vi "One shot TCP AI.vi"() -> ()   [LabVIEW 2010]
uses:
  Send 1 Scan multi-channel.vi
  scale.ctl
  DAQ configuration/channel identifier.ctl
panel:
  in  "Reset graph":bool
  in  "history length":u16=1000 min=1
  out "XY Graph":cluster{dbl[], dbl[]}[](graph)
  out "Range error":bool[](array[boolean])
  out "units":string[](array[string])
  out "Scaled data":sgl[](array[numeric]) format="%.2f"
  out "voltage date":sgl[](array[numeric]) format="%.5f"
  in  "Scale type":T1[](array[typedef]) items=["200 kPa - cm", "200 kPa - orifice 1.6 mm", "200 kPa - orifice 3.2 mm", "200 kPa - Pa", "7 kPa - 1.5 cm vol det", "7 kPa - 10 cm vol det", "7 kPa - cm", "7 kPa - orifice 1.6 mm", "7 kPa - orifice 3.2 mm", "7 kPa - Pa", "7 kPa - Reservoir", "Thermistors - C1", "Thermistors - C2", "Thermistors - C3", "Thermistors - C4", "Thermistors - C5", "Thermistors - C6", "Thermistors - C7"]
  in  "Port":T2[](array[typedef])
  out "arbitrary time (s)":dbl format="%.2f"
  in  "millisecond multiple":u32
  in  "stop":bool
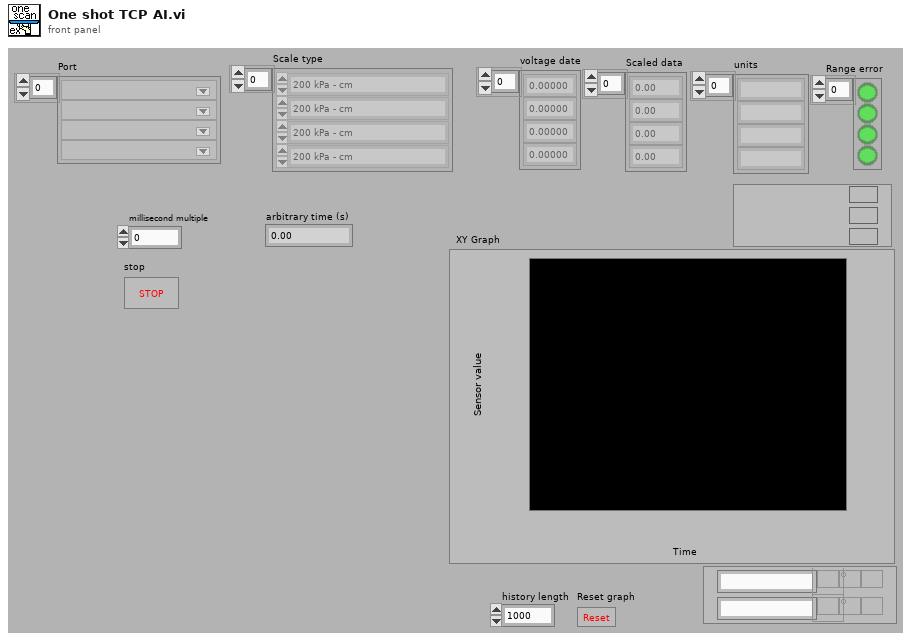
[diagram p1: front panel]
types:
  T1 = typedef "scale.ctl" = u16
  T2 = typedef "channel identifier.ctl" = u16
  T3 = cluster{"scan rate":dbl, "# connections":i32, "channels (0)":string[], "group channel settings":cluster{"channel":string, "upper input limits":sgl, "lower input limits":sgl, "range":sgl, "polarity":enum16{"no change", "bipolar", "unipolar"}, "gain":sgl, "coupling":enum16{"no change", "DC", "AC", "ground", "internal reference"}, "input mode":enum16{"no change", "differential", "rse", "nrse"}, "scale multiplier":sgl, "scale offset":sgl}[]}
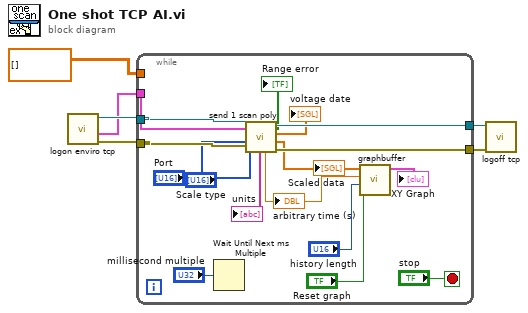
[diagram p0: block diagram]
diagram:
  n1 = call "logon enviro tcp.vi"(1:w2) -> ("error out"=w4:errorcluster, "connection ID"=w5:refnum<k5>)  [unwired: 8 in, 1 out]
  n2 = while {
    tunnel: [w16] -> w2
    tunnel: sgl[][] [] ("History Data") -> [_]
    tunnel: [w18] -> w3
    tunnel: w4 -> [w21]
    tunnel: w5 -> [w22]
    tunnel: [w23] -> w6
    stop <- "stop" stop-if-true
    n3 = Wait Until Next ms Multiple(millisecond multiple="millisecond multiple") -> ()  [unwired: 1 out]
    n4 = call-poly "send 1 scan poly.vi"("error in (no error)"=w21, "Scale type"="Scale type", "Port"="Port", "Connection ID in"=w22) -> ("error out"=w23:errorcluster, "Scaled data"=w10:sgl[], "voltage data"=→"voltage date":sgl[], "Connection ID out"=w18:refnum<k5>, "arbitrary time (s)"=w17:dbl, "Out of Range"=→"Range error":bool[], "units"=→"units":string[], "Server Stats"=w16:T3)
    "arbitrary time (s)" <- w17
    "Scaled data" <- w10
    n5 = call "graphbuffer.vi"("Reset"="Reset graph", "history length"="history length", "Time"=w17, "data"=w10) -> ("Multiplot graph data"=→"XY Graph":cluster{dbl[], dbl[]}[])  [unwired: 5 in, 2 out]
  }
  n6 = call "logoff tcp.vi"("error in (no error)"=w6, "Connection ID"=w3) -> ()  [unwired: 8 in, 2 out]
